vi "Main.vi"() -> ()   [LabVIEW 2026]
doc: "This template is for the Queued Message Handler design pattern.\n\nThe Event Handling Loop generates messages based on user interface actions.\n\nThe Message Handling Loop processes messages generated by the Event Handling Loop, or by other messages. The messages are string values, so new messages can be added easily to the Message Cases case structure in the Message Handling Loop. Each message cluster can also provide an optional value for Message Data, which is a variant that can be converted to whatever message-specific data is required."
uses:
  SubVIs/Controls/PCO_Config.ctl
  SubVIs/Controls/UI Data.ctl
  <instrlib>/PCO_SDK/File Group 0/vi.lib/Excelitas PCO GmbH/pco.labview/camera/Camera.lvclass
  SubVIs/Controls/TypeDef_FGV.ctl
  SubVIs/QMH/Message Queue/Enqueue Message (Single).vi
  SubVIs/QMH/Message Queue/Message Queue.lvlib
  SubVIs/QMH/User Event - Stop/User Event - Stop.lvlib
  <instrlib>/PCO_SDK/File Group 0/vi.lib/Excelitas PCO GmbH/pco.labview/pco.sdk/TimingControl/TimingControl.lvlib
panel:
  in  "# of frames":u16=10
  in  "SavePath":path
  out "Camera":u16[][](graph)
  in  "Stop live":bool
  in  "Grab":bool
  in  "Live":bool
  in  "PCO_Config":T1={"Exposure time (s)"=0.1, "TriggerMode"=0, "ROI X0"=1, "ROI Y0"=1, "ROI X1"=2048, "ROI Y1"=2048, "Binning"=1} {"TriggerMode" items=["auto sequence", "software trigger", "external exposure start", "external exposure control"]}
  out "Current task":string="\"Exit\" button pressed"
  in  "Exit":bool
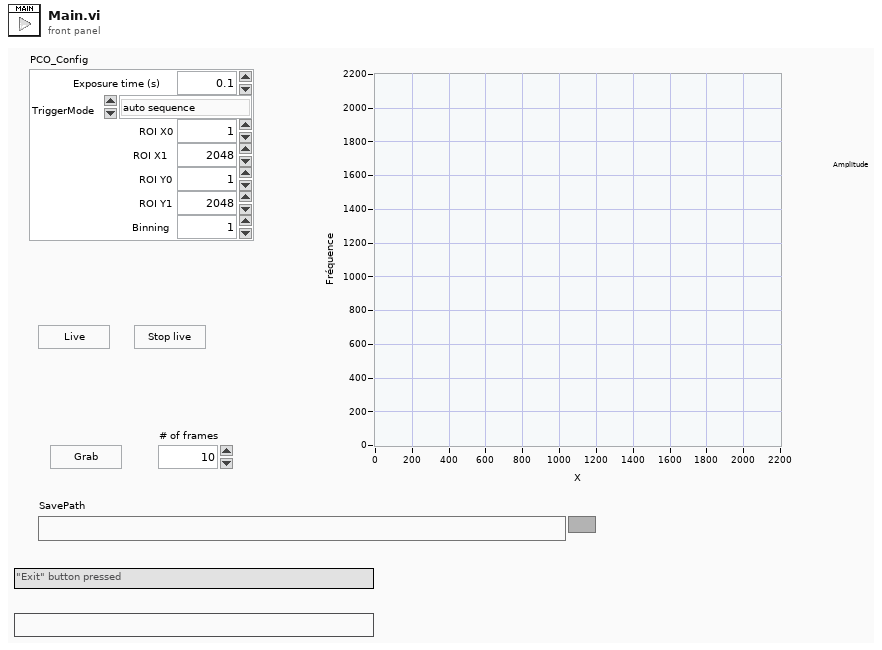
[diagram p1: front panel]
types:
  T1 = typedef "PCO_Config.ctl" = cluster{"Exposure time (s)":dbl, "TriggerMode":u16, "ROI X0":u16, "ROI Y0":u16, "ROI X1":u16, "ROI Y1":u16, "Binning":u8}
  T2 = typedef "UI Data.ctl" = cluster{"Data Display Ref":refnum<vi>, "Exit Button Ref":refnum<vi>, "Message":string}
  T3 = typedef "Message Queue.lvlib/All Message Queues.ctl" = cluster{"UI":refnum<queue>, "Camera loop":refnum<queue>, "Display loop":refnum<queue>}
  T4 = typedef "TypeDef_FGV.ctl" = enum16{"Initialize", "Write", "Read"}
  T5 = typedef "Camera.lvclass/binning.ctl" = cluster{"vert":u16, "horz":u16, "mode":u16}
  T6 = cluster{"exposure_time_s":dbl, "delay_time_s":dbl, "roi":cluster{"x0":u64, "y0":u64, "x1":u64, "y1":u64}, "timestamp_mode":u16, "pixelrate":u32, "trigger_mode":u16, "acquire_mode":u16, "metadata_mode":u16, "noisefilter_mode":u16, "pixel_format":u32, "binning":T5, "auto_exposure":cluster{"region":u16, "min_exposure_s":dbl, "max_exposure_s":dbl}}
  T7 = cluster{"wSignalNum":u16, "wEnabled":u16, "wType":u16, "wPolarity":u16, "wFilterSetting":u16, "wSelected":u16, "dwParameter":u32[], "dwSignalFunctionality":u32[]}
  T8 = cluster{"wVersion":u16, "dwIMAGE_COUNTER":u32, "dwIMAGE_TIME_US":u32, "lvTimestamp":timestamp, "bIMAGE_TIME_STATUS":u8, "wEXPOSURE_TIME_BASE":u16, "dwEXPOSURE_TIME":u32, "dwFRAMERATE_MILLIHZ":u32, "sSENSOR_TEMPERATURE":i16, "wIMAGE_SIZE_X":u16, "wIMAGE_SIZE_Y":u16, "bBINNING_X":u8, "bBINNING_Y":u8, "dwSENSOR_READOUT_FREQUENCY":u32, "wSENSOR_CONV_FACTOR":u16, "dwCAMERA_SERIAL_NO":u32, "wCAMERA_TYPE":u16, "bBIT_RESOLUTION":u8, "bSYNC_STATUS":u8, "wDARK_OFFSET":u16, "bTRIGGER_MODE":u8, "bDOUBLE_IMAGE_MODE":u8, "bCAMERA_SYNC_MODE":u8, "bIMAGE_TYPE":u8, "wCOLOR_PATTERN":u16, "wCAMERA_SUBTYPE":u16, "dwEVENT_NUMBER":u32, "wIMAGE_SIZE_X_Offset":u16, "wIMAGE_SIZE_Y_Offset":u16, "bREADOUT_MODE":u8}[]
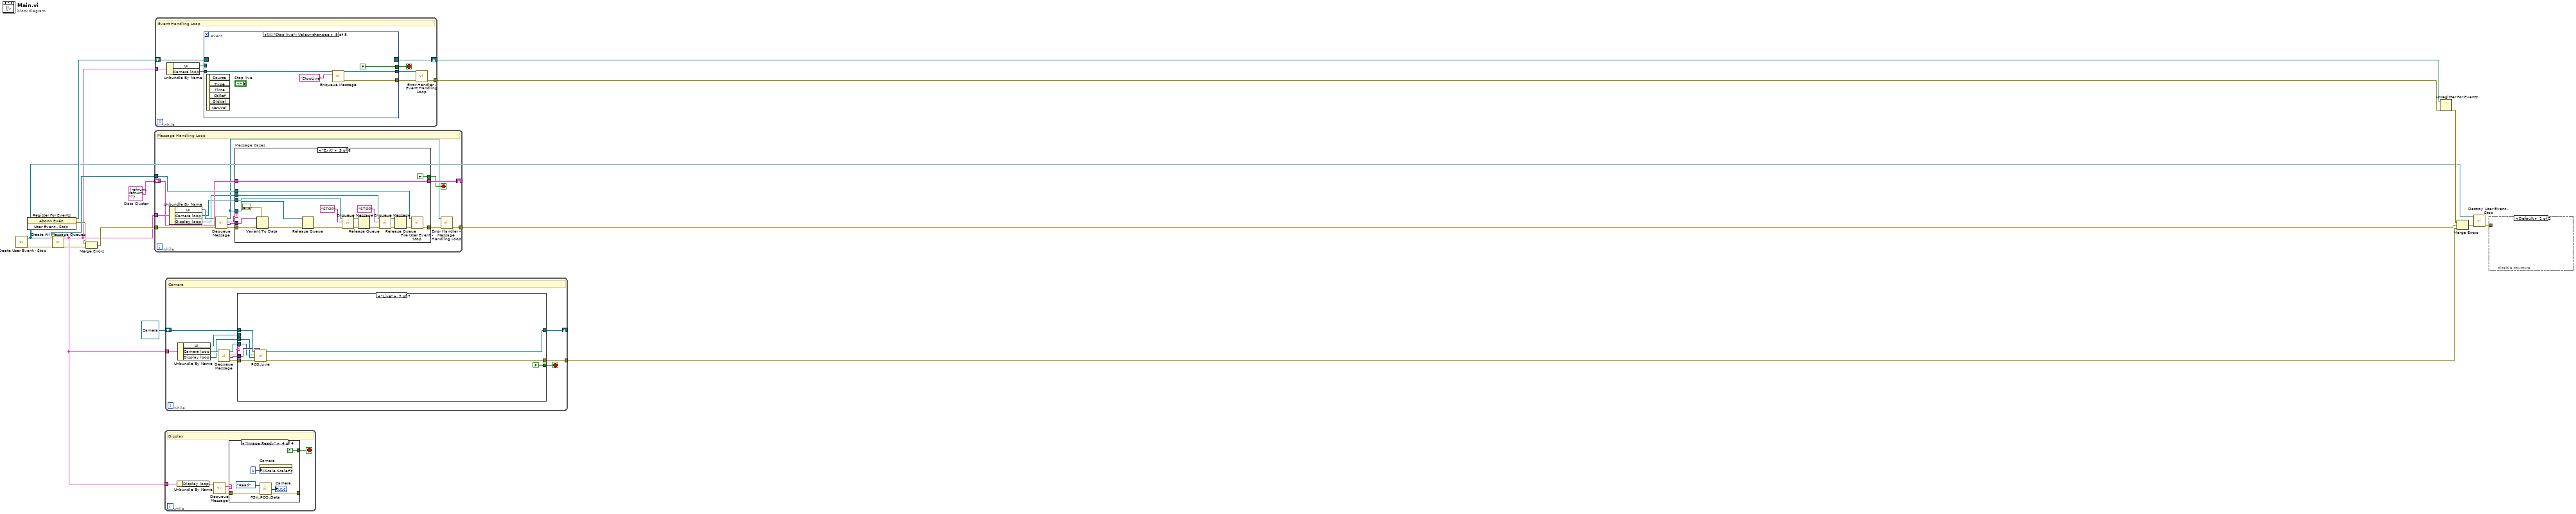
[diagram p0: block diagram]
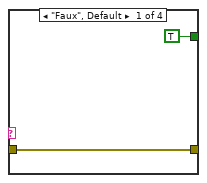
[diagram p2: hidden frame]
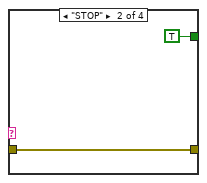
[diagram p3: hidden frame]
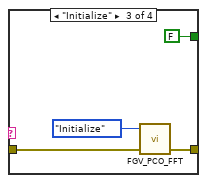
[diagram p4: hidden frame]
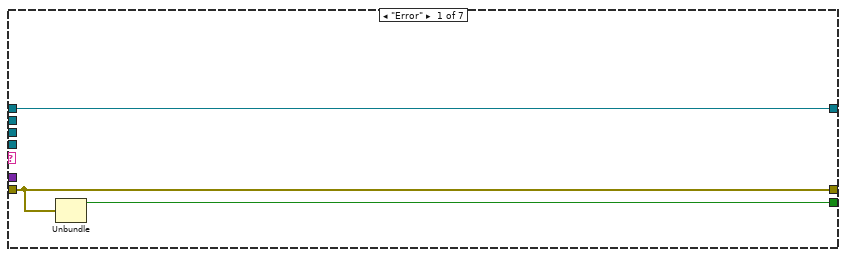
[diagram p5: hidden frame]
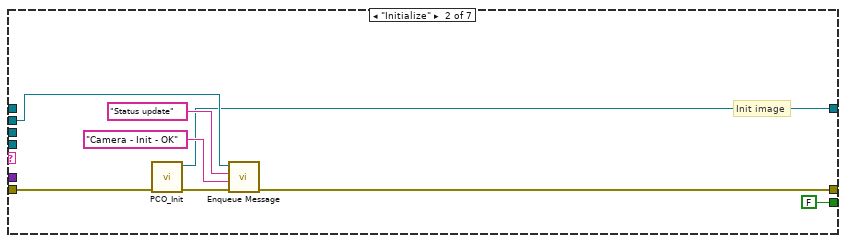
[diagram p6: hidden frame]
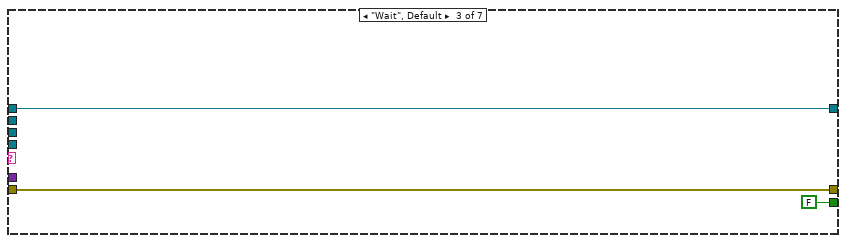
[diagram p7: hidden frame]
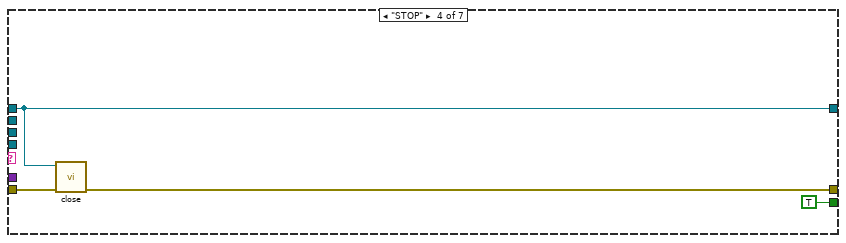
[diagram p8: hidden frame]
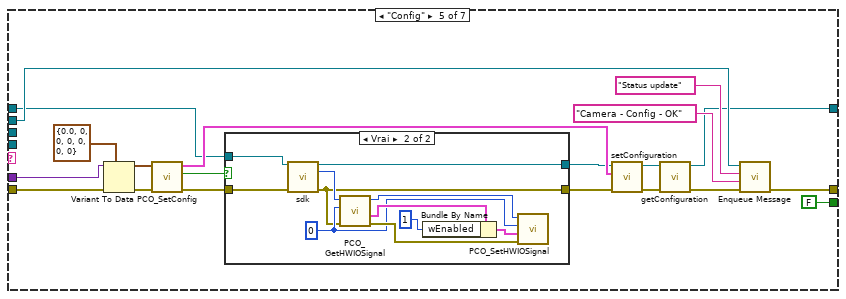
[diagram p9: hidden frame]
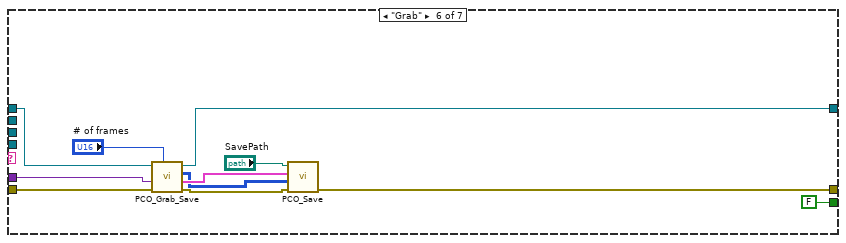
[diagram p11: hidden frame]
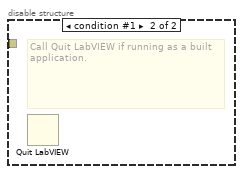
[diagram p12: hidden frame]
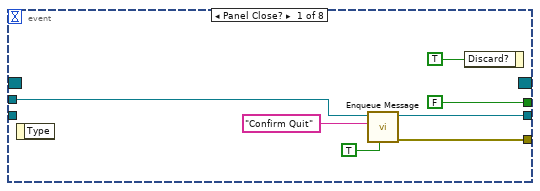
[diagram p13: hidden frame]
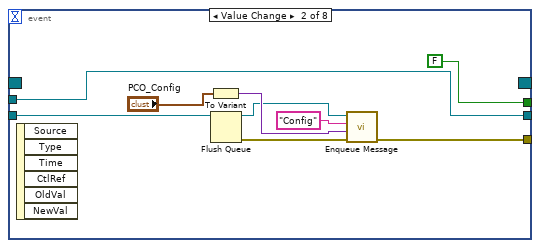
[diagram p14: hidden frame]
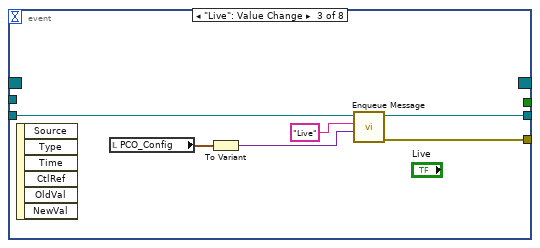
[diagram p15: hidden frame]
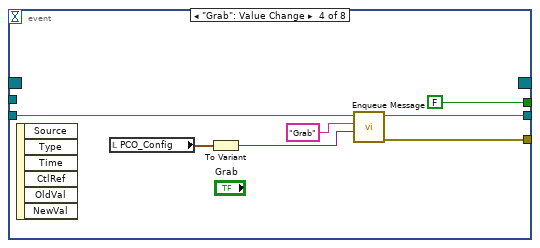
[diagram p16: hidden frame]
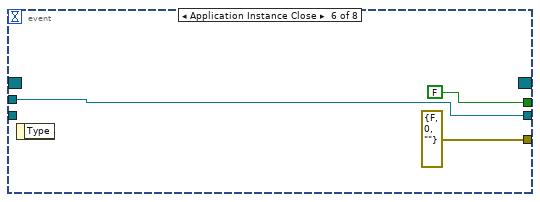
[diagram p17: hidden frame]
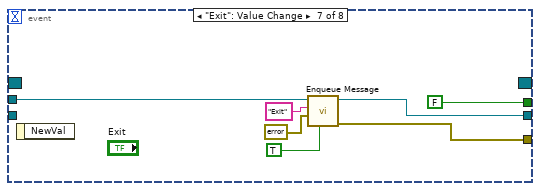
[diagram p18: hidden frame]
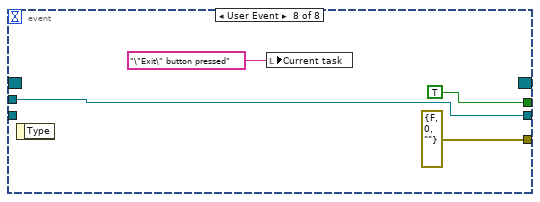
[diagram p19: hidden frame]
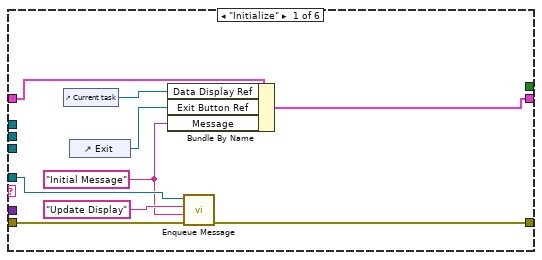
[diagram p20: hidden frame]
diagram:
  w4 = T2 {"Data Display Ref"=refnum, "Exit Button Ref"=refnum, "Message"=""}  # Data Cluster
  n1 = call "Create User Event - Stop.vi"() -> ("error out"=w14:errorcluster, "User Event - Stop"=w7:refnum<user-event>)  [unwired: 10 in]
  n2 = register-events(w7) -> (reference out=w8:refnum<event-registration>, error out=w5:errorcluster)  [unwired: 2 in]
  n3 = call "Create All Message Queues.vi"("error in (no error)"=w14) -> ("error out"=w16:errorcluster, "Message Queues out"=w2:T3)  [unwired: 9 in]
  n4 = Merge Errors(w5, w16) -> (w6:errorcluster)
  n5 = while {
    shift-right: [w30] -> _
    shift-left: w4 -> [w31]
    tunnel: w7 -> [w28]
    tunnel: w6 -> [w27]
    tunnel: [w22] -> w15
    tunnel: w2 -> [w20]
    stop <- w29 stop-if-true
    # "Message Handling Loop"
    n6 = Unbundle By Name(w20) -> ("UI"=w19:refnum<queue>, "Camera loop"=w18:refnum<queue>, "Display loop"=w17:refnum<queue>)
    n7 = call "Dequeue Message.vi"("error in (no error)"=w27, "Message Queue"=w19) -> ("error out"=w26:errorcluster, "Message Data"=w24:variant, "Message"=w25:string, "dup Message Queue"=w23:refnum<queue>)  [unwired: 6 in]
    n8 = case "Message Cases" shown="\"Exit\"" w25 {
      tunnel: w23 -> [w34 _ _ w56 w70 _]
      tunnel: w26 -> [w39 w45 w52 w58 w71 w79]
      tunnel: [w40 w42 w47 w53 w66 w79] -> w21
      tunnel: w31 -> [w38 w46 w51 w57 w78 w80]
      tunnel: [w37 w46 w51 w57 w78 w80] -> w30
      tunnel: [_ _ _ _ TRUE _] -> w29
      tunnel: w24 -> [_ w44 w50 _ w74 _]
      tunnel: w28 -> [_ _ _ _ w76 _]
      tunnel: w18 -> [_ _ _ _ w69 _]
      tunnel: w17 -> [_ _ _ _ w59 _]
      frame "Initialize" {
        w32 = "Initial Message" ("Initial Message")
        n9 = control-ref of="Current task"() -> (w33:refnum<vi>)
        n10 = control-ref of="Exit"() -> (w36:refnum<vi>)
        n11 = Bundle By Name(cluster=w38, "Data Display Ref"=w33, "Exit Button Ref"=w36, "Message"=w32) -> (w37:T2)
        n12 = call-poly "Enqueue Message.vi"("error in (no error)"=w39, "Message Data"=w32, "Message"="Update Display", "Message Queue"=w34) -> ("error out"=w40:errorcluster)  [unwired: 6 in, 1 out]
      }
      frame "Update Display" {
        n13 = Variant To Data(error in=w45, type="", Variant=w44) -> (data=→"Current task":string, error out=w42:errorcluster)
      }
      frame "Error" {
        n14 = Variant To Data(error in=w52, type=errorcluster {"status"=FALSE, "code"=0, "source"=""} ("error constant"), Variant=w50) -> (data=w48:errorcluster, error out=w47:errorcluster)
        n15 = call <vilib>:"Simple Error Handler.vi"("error in (no error)"=w48) -> ()  [unwired: 4 in, 5 out]
      }
      frame "Confirm Quit" {
        n16 = call-poly "Enqueue Message.vi"("Priority Message? (F)"=TRUE, "error in (no error)"=w58, "Message"="Exit", "Message Queue"=w56) -> ("error out"=w53:errorcluster)  [unwired: 6 in, 1 out]
      }
      frame "Exit" {
        n17 = Variant To Data(error in=w71, type=errorcluster {"status"=FALSE, "code"=0, "source"=""} ("error constant"), Variant=w74) -> (error out=w67:errorcluster)  [unwired: 1 out]
        n18 = Release Queue(queue=w70, error in (no error)=w67) -> (error out=w65:errorcluster)  [unwired: 1 in, 2 out]
        n19 = call-poly "Enqueue Message.vi"("error in (no error)"=w65, "Message"="STOP", "Message Queue"=w69) -> ("error out"=w73:errorcluster, "dup Message Queue"=w72:refnum<queue>)  [unwired: 7 in]
        n20 = Release Queue(queue=w72, error in (no error)=w73) -> (error out=w61:errorcluster)  [unwired: 1 in, 2 out]
        n21 = call-poly "Enqueue Message.vi"("error in (no error)"=w61, "Message"="STOP", "Message Queue"=w59) -> ("error out"=w62:errorcluster, "dup Message Queue"=w63:refnum<queue>)  [unwired: 7 in]
        n22 = Release Queue(queue=w63, error in (no error)=w62) -> (error out=w60:errorcluster)  [unwired: 1 in, 2 out]
        n23 = call "Fire User Event - Stop.vi"("error in (no error)"=w60, "User Event - Stop"=w76) -> ("error out"=w66:errorcluster)  [unwired: 9 in]
      }
      frame Default {
      }
    }
    n24 = call "Error Handler - Message Handling Loop.vi"("error in (no error)"=w21, "Message Queue"=w23) -> ("dup error in"=w22:errorcluster)  [unwired: 8 in, 1 out]
  }
  n25 = while {
    shift-right: [w88] -> w11
    shift-left: w8 -> [w89]
    tunnel: [w84] -> w9
    tunnel: w2 -> [w81]
    stop <- w86 stop-if-true
    # "Event Handling Loop"
    n26 = Unbundle By Name(w81) -> ("UI"=w83:refnum<queue>, "Camera loop"=w82:refnum<queue>)
    n27 = event shown="[4] \"Stop live\": Valeur changée" {
      selector: w89 -> [_ _ _ _ _ _ _ _]
      dyn-events: [_ _ _ _ _ _ _ _] -> w88
      timeout: _ -> [_ _ _ _ _ _ _ _]
      tunnel: [FALSE ("Discard?") FALSE ("Discard?") _ FALSE ("Discard?") FALSE ("Discard?") FALSE ("Discard?") FALSE ("Discard?") TRUE ("Discard?")] -> w86
      tunnel: w83 -> [w95 w105 _ _ _ w126 w133 w137]
      tunnel: [w94 w101 w108 w115 w121 errorcluster {"status"=FALSE, "code"=0, "source"=""} ("error out") w127 errorcluster {"status"=FALSE, "code"=0, "source"=""} ("error out")] -> w87
      tunnel: [w93 w105 w107 w116 w120 w126 w132 w137] -> w85
      tunnel: w82 -> [_ w99 w106 w117 w122 _ _ _]
      event Panel Close? {
        n28 = event-data() -> ()  [unwired: 1 in, 1 out]
        n29 = call-poly "Enqueue Message.vi"("Priority Message? (F)"=TRUE, "Message"="Confirm Quit", "Message Queue"=w95) -> ("error out"=w94:errorcluster, "dup Message Queue"=w93:refnum<queue>)  [unwired: 7 in]
        n30 = event-data("Discard?"=TRUE) -> ()  [unwired: 1 in, 1 out]
      }
      event Value Change {
        n31 = event-data() -> ()  [unwired: 1 in, 6 out]
        n32 = To Variant(anything="PCO_Config") -> (Variant=w102:variant)
        n33 = Flush Queue(queue=w99) -> (queue out=w97:refnum<queue>, error out=w98:errorcluster)  [unwired: 1 in, 1 out]
        n34 = call-poly "Enqueue Message.vi"("error in (no error)"=w98, "Message Data"=w102, "Message"="Config", "Message Queue"=w97) -> ("error out"=w101:errorcluster)  [unwired: 6 in, 1 out]
      }
      event "Live": Value Change {
        n35 = event-data() -> ()  [unwired: 1 in, 6 out]
        n36 = local read "PCO_Config"() -> (w111:T1)
        n37 = To Variant(anything=w111) -> (Variant=w110:variant)
        n38 = call-poly "Enqueue Message.vi"("Message Data"=w110, "Message"="Live", "Message Queue"=w106) -> ("error out"=w108:errorcluster, "dup Message Queue"=w107:refnum<queue>)  [unwired: 7 in]
      }
      event "Grab": Value Change {
        n39 = event-data() -> ()  [unwired: 1 in, 6 out]
        n40 = local read "PCO_Config"() -> (w113:T1)
        n41 = To Variant(anything=w113) -> (Variant=w112:variant)
        n42 = call-poly "Enqueue Message.vi"("Message Data"=w112, "Message"="Grab", "Message Queue"=w117) -> ("error out"=w115:errorcluster, "dup Message Queue"=w116:refnum<queue>)  [unwired: 7 in]
      }
      event "Stop live": Value Change {
        n43 = event-data() -> ()  [unwired: 1 in, 6 out]
        n44 = call-poly "Enqueue Message.vi"("Message"="StopLive", "Message Queue"=w122) -> ("error out"=w121:errorcluster, "dup Message Queue"=w120:refnum<queue>)  [unwired: 8 in]
      }
      event Application Instance Close {
        n45 = event-data() -> ()  [unwired: 1 in, 1 out]
      }
      event "Exit": Value Change {
        n46 = event-data() -> ()  [unwired: 1 in, 1 out]
        n47 = call-poly "Enqueue Message.vi"("Priority Message? (F)"=TRUE, "Message Data"=errorcluster {"status"=FALSE, "code"=0, "source"=""} ("error constant"), "Message"="Exit", "Message Queue"=w133) -> ("error out"=w127:errorcluster, "dup Message Queue"=w132:refnum<queue>)  [unwired: 6 in]
      }
      event User Event {
        n48 = event-data() -> ()  [unwired: 1 in, 1 out]
        n49 = local write "Current task"("\"Exit\" button pressed" ("VI Stopped")) -> ()
      }
    }
    n50 = call "Error Handler - Event Handling Loop.vi"("error in (no error)"=w87, "Message Queue"=w85) -> ("dup error in"=w84:errorcluster)  [unwired: 8 in, 1 out]
  }
  n51 = while {
    tunnel: w2 -> [w142]
    stop <- w138 stop-if-true
    # "Display"
    n52 = Unbundle By Name(w142) -> ("Display loop"=w141:refnum<queue>)
    n53 = call "Dequeue Message.vi"("Message Queue"=w141) -> ("error out"=w139:errorcluster, "Message"=w140:string)  [unwired: 7 in, 2 out]
    n54 = case shown="\"Image Ready\"" w140 {
      tunnel: w139 -> [w144 w145 w149 w155]
      tunnel: [w144 w145 w148 w153] -> _
      tunnel: [TRUE TRUE FALSE FALSE] -> w138
      frame "Faux", Default {
      }
      frame "STOP" {
      }
      frame "Initialize" {
        n55 = call "FGV_PCO_FFT.vi"("error in"=w149, "Action"=TypeDef_FGV."Initialize") -> ("error out"=w148:errorcluster)  [unwired: 2 in, 1 out]
      }
      frame "Image Ready" {
        n56 = property on="Camera" class="GraphInt (strict)"("ZScale.ScaleFit"=u8 1 ("Échelle des Z.Ajuster l'échelle")) -> ()  [unwired: 2 in, 2 out]
        n57 = call "FGV_PCO_Data.vi"("error in"=w155, "Action"=TypeDef_FGV."Read") -> ("error out"=w153:errorcluster, "Data"=→"Camera":u16[][])  [unwired: 2 in]
      }
    }
  }
  n58 = while {
    tunnel: [w164] -> w3
    tunnel: w2 -> [w163]
    shift-right: [w161] -> _
    shift-left: refnum<class "Camera.lvclass"> refnum ("Camera out") -> [w160]
    stop <- w165 stop-if-true
    # "Camera"
    n59 = Unbundle By Name(w163) -> ("UI"=w162:refnum<queue>, "Camera loop"=w159:refnum<queue>, "Display loop"=w158:refnum<queue>)
    n60 = call "Dequeue Message.vi"("Message Queue"=w159) -> ("error out"=w168:errorcluster, "Message Data"=w166:variant, "Message"=w167:string, "dup Message Queue"=w157:refnum<queue>)  [unwired: 7 in]
    n61 = case shown="\"Live\"" w167 {
      tunnel: w168 -> [w171 w175 w182 w185 w205 w227 w236]
      tunnel: w166 -> [_ _ _ _ w204 w226 w235]
      tunnel: w162 -> [_ w179 _ _ w199 _ _]
      tunnel: [w170 FALSE ("status") FALSE ("status") TRUE FALSE ("status") FALSE ("status") FALSE ("status")] -> w165
      tunnel: [w171 w173 w182 w184 w198 w220 w233] -> w164
      tunnel: w157 -> [_ _ _ _ _ _ w231]
      tunnel: [w169 w174 w181 w183 w193 w230 w232] -> w161
      tunnel: w160 -> [w169 _ w181 w183 w191 w225 w237]
      tunnel: w158 -> [_ _ _ _ _ _ w234]
      frame "Error" {
        n62 = Unbundle(w171) -> ("status"=w170:bool)  [unwired: 2 out]
      }
      frame "Initialize" {
        # "Init image"
        n63 = call "PCO_Init.vi"("entrée d'erreur (pas d'erreur)"=w175) -> ("sortie d'erreur"=w172:errorcluster, "Camera en sortie"=w174:refnum<class "Camera.lvclass">)  [unwired: 9 in]
        n64 = call-poly "Enqueue Message.vi"("error in (no error)"=w172, "Message Data"="Camera - Init - OK", "Message"="Status update", "Message Queue"=w179) -> ("error out"=w173:errorcluster)  [unwired: 6 in, 1 out]
      }
      frame "Wait", Default {
      }
      frame "STOP" {
        n65 = call-dynamic "close.vi"("error in (no error)"=w185, "Camera in"=w183) -> ("error out"=w184:errorcluster)  [unwired: 9 in]
      }
      frame "Config" {
        n66 = Variant To Data(error in=w205, type=T1 {"Exposure time (s)"=0.0, "TriggerMode"=0, "ROI X0"=0, "ROI Y0"=0, "ROI X1"=0, "ROI Y1"=0, "Binning"=0} ("PCO_Config"), Variant=w204) -> (data=w202:T1, error out=w188:errorcluster)
        n67 = call "PCO_SetConfig.vi"("error in"=w188, "PCO_Config"=w202) -> ("error out"=w187:errorcluster, "Trigger externe?"=w189:bool, "configuration"=w201:T6)  [unwired: 7 in]
        n68 = case shown="Vrai" w189 {
          tunnel: w187 -> [w208 w212]
          tunnel: [w208 w211] -> w192
          tunnel: w191 -> [w207 w210]
          tunnel: [w207 w209] -> w190
          frame False {
          }
          frame True {
            w214 = u16 0 ("wSignalNum")
            n69 = call-dynamic "sdk.vi"("Camera in"=w210, "error in (no error)"=w212) -> ("Camera out"=w209:refnum<class "Camera.lvclass">, "sdk"=w215:u64, "error out"=w211:errorcluster)  [unwired: 11 in]
            n70 = call <instrlib>:"PCO_GetHWIOSignal.vi"("error in (no error)"=w211, "wSignalNum"=w214, "ph"=w215) -> ("error out"=w217:errorcluster, "strSignal"=w219:T7, "ph out"=w216:u64)  [unwired: 5 in, 1 out]
            n71 = Bundle By Name(cluster=w219, "wEnabled"=u16 1) -> (w218:T7)
            n72 = call <instrlib>:"PCO_SetHWIOSignal.vi"("error in (no error)"=w217, "strSignal"=w218, "wSignalNum"=w214, "ph"=w216) -> ()  [unwired: 5 in, 3 out]
          }
        }
        n73 = call-dynamic "setConfiguration.vi"("error in (no error)"=w192, "configuration"=w201, "Camera in"=w190) -> ("error out"=w194:errorcluster, "Camera out"=w195:refnum<class "Camera.lvclass">)  [unwired: 7 in]
        n74 = call-dynamic "getConfiguration.vi"("error in (no error)"=w194, "Camera in"=w195) -> ("error out"=w196:errorcluster, "Camera out"=w193:refnum<class "Camera.lvclass">)  [unwired: 7 in, 1 out]
        n75 = call-poly "Enqueue Message.vi"("error in (no error)"=w196, "Message Data"="Camera - Config - OK", "Message"="Status update", "Message Queue"=w199) -> ("error out"=w198:errorcluster)  [unwired: 6 in, 1 out]
      }
      frame "Grab" {
        n76 = call "PCO_Grab_Save.vi"("# of frames"="# of frames", "entrée d'erreur (pas d'erreur)"=w227, "Message Data"=w226, "Camera en entrée"=w225) -> ("sortie d'erreur"=w223:errorcluster, "meta_data_list"=w222:T8, "Raw data (U16)"=w221:u16[][][], "Camera en sortie"=w230:refnum<class "Camera.lvclass">)  [unwired: 4 in]
        n77 = call "PCO_Save.vi"("entrée d'erreur (pas d'erreur)"=w223, "raw_image_list (U16)"=w221, "meta_data_list"=w222, "SavePath"="SavePath") -> ("sortie d'erreur"=w220:errorcluster)  [unwired: 7 in]
      }
      frame "Live" {
        n78 = call "PCO_Live.vi"("Message Data"=w235, "entrée d'erreur (pas d'erreur)"=w236, "Display loop"=w234, "dup Message Queue"=w231, "Camera en entrée"=w237) -> ("sortie d'erreur"=w233:errorcluster, "Camera en sortie"=w232:refnum<class "Camera.lvclass">)  [unwired: 5 in]
      }
    }
  }
  n79 = Unregister For Events(event registration refnum=w11, error in=w9) -> (error out=w12:errorcluster)
  n80 = Merge Errors(w12, w15, w3) -> (w13:errorcluster)
  n81 = call "Destroy User Event - Stop.vi"("error in (no error)"=w13, "User Event - Stop"=w7) -> ("error out"=w10:errorcluster)  [unwired: 9 in]
  n82 = disable-structure shown="Default" {
    disable-tunnel: w10 -> [_ _]
    frame condition #0 (active) {
    }
    frame condition #1 {
      # "Call Quit LabVIEW if running as a built application."
      n83 = Quit LabVIEW() -> ()  [unwired: 1 in]
    }
  }
